vi "Get Project Paths.vi"(8 "error in (no error)":errorcluster, 10 "Name":string, 11 "ProjectItem refnum":refnum<vi>) -> (0 "error out":errorcluster, 1 "Virtual Path":string[](array[string]), 3 "Path on Disk":path[](array[path]))   [LabVIEW 2023]
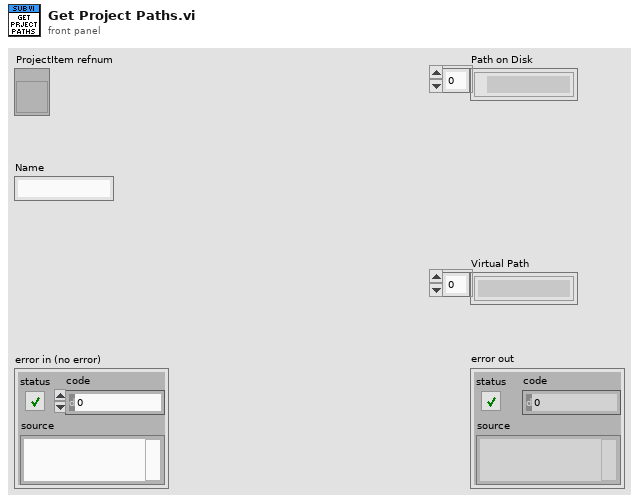
[diagram p1: front panel]
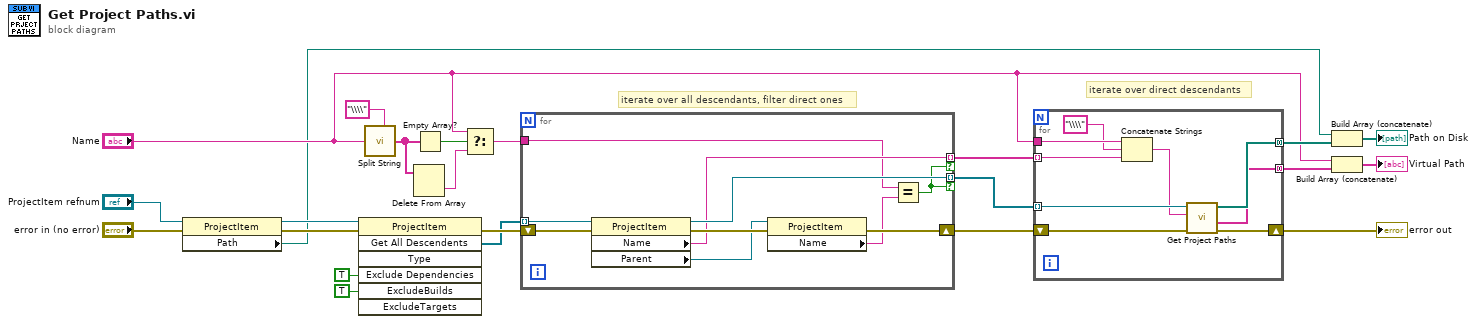
[diagram p0: block diagram]
diagram:
  # "iterate over all descendants, filter direct ones"
  # "iterate over direct descendants"
  n1 = property class="ProjectItem"(reference="ProjectItem refnum", error in="error in (no error)") -> (reference out=w8:refnum<vi>, error out=w9:errorcluster, "Path"=w1:path)
  n2 = invoke class="ProjectItem" method="Get All Descendents"(reference=w8, error in=w9, "Exclude Dependencies"=TRUE ("ExcludeDependencies"), "ExcludeBuilds"=TRUE) -> (error out=w23:errorcluster, "All Descendents"=w22:refnum<vi>[])  [unwired: 3 in, 5 out]
  n3 = call <vilib>:"Split String.vi"("Split Pattern"="\\\\", "Input String"="Name") -> ("Split String"=w12:string[])  [unwired: 5 in]
  n4 = Delete From Array(array=w12) -> (deleted portion=w11:string)  [unwired: 2 in, 1 out]
  n5 = Empty Array?(array=w12) -> (empty?=w13:bool)
  n6 = Select(t="Name", s=w13, f=w11) -> (s? t:f=w10:string)
  n7 = for {
    tunnel: w22 -> [w30] mode=indexing
    tunnel: w10 -> [w24]
    tunnel: [w27] -> w19 mode=indexing if=w25
    tunnel: [w26] -> w17 mode=indexing if=w25
    shift-right: [w31] -> w4
    shift-left: w23 -> [w33]
    n8 = property class="ProjectItem"(reference=w30, error in=w33) -> (reference out=w27:refnum<vi>, error out=w32:errorcluster, "Name"=w26:string, "Parent"=w29:refnum<vi>)
    n9 = property class="ProjectItem"(reference=w29, error in=w32) -> (error out=w31:errorcluster, "Name"=w28:string)  [unwired: 1 out]
    n10 = Equal?(x=w24, y=w28) -> (x = y?=w25:bool)
  }
  n11 = for {
    tunnel: w19 -> [w42] mode=indexing
    tunnel: [w41] -> w18 mode=concatenating
    tunnel: w17 -> [w37] mode=indexing
    tunnel: [w40] -> w16 mode=concatenating
    tunnel: "Name" -> [w39]
    shift-right: [w34] -> w3
    shift-left: w4 -> [w35]
    n12 = Concatenate Strings(w39, "\\\\" ("string"), w37) -> (w38:string)
    n13 = call "Get Project Paths.vi"("error in (no error)"=w35, "Name"=w38, "ProjectItem refnum"=w42) -> ("error out"=w34:errorcluster, "Virtual Path"=w40:string[], "Path on Disk"=w41:path[])  [unwired: 6 in]
  }
  "error out" <- w3
  n14 = Build Array (concatenate)(w1, w18) -> (→"Path on Disk":path[])
  n15 = Build Array (concatenate)("Name", w16) -> (→"Virtual Path":string[])
